vi "Write error details.vi"(8 "error in (no error)":errorcluster, 10 "error details":errorcluster, 11 "Printer_ZEBRA in":refnum<class "Printer_ZEBRA.lvclass">) -> (0 "error out":errorcluster, 3 "Printer_ZEBRA out":refnum<class "Printer_ZEBRA.lvclass">)   [LabVIEW 2021, in "Printer_ZEBRA.lvclass"]
uses:
  Printer_ZEBRA.lvclass
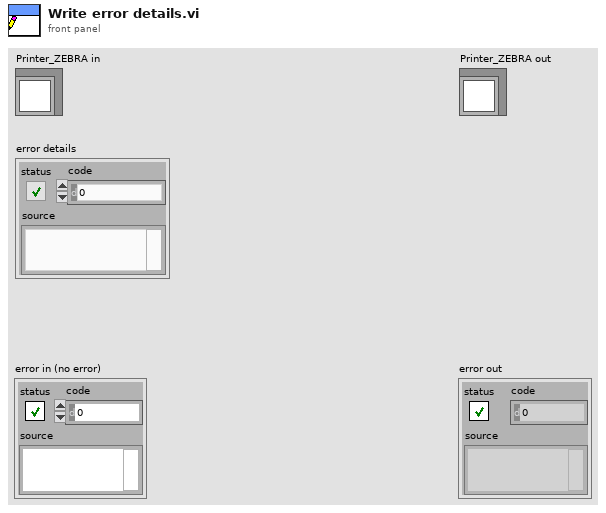
[diagram p1: front panel]
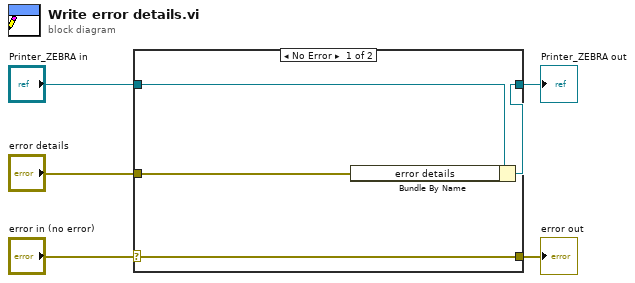
[diagram p0: block diagram]
diagram:
  n1 = case shown="No Error" "error in (no error)" {
    selector: "error in (no error)" -> [w9 w10]
    tunnel: [w9 w10] -> w4
    tunnel: [w7 w11] -> w2
    tunnel: "Printer_ZEBRA in" -> [w8 w11]
    tunnel: "error details" -> [w6 _]
    frame No Error {
      n2 = Bundle By Name(cluster=w8, "error details"=w6) -> (w7:refnum<class "Printer_ZEBRA.lvclass">)
    }
    frame Error {
    }
  }
  "error out" <- w4
  "Printer_ZEBRA out" <- w2
